vi "RL-Spect-Fast.vi"() -> ()   [LabVIEW 2014]
doc: "Random Laser Project\n\nAndré Romero - 2020\nandretec@ifsc.usp.br\n\nMain Program"
uses:
  Global variables.vi
panel:
  in  "Integration Time":i32=100
  in  "Average":i32=1
  out "Delay Power Meter":u32
  out "Delay Spectrum":u32
  in  "Stop Button":bool
  out "Power":dbl
  in  "Average Time (0.0)":dbl=0.1
  out "XY Graph":T1(graph)
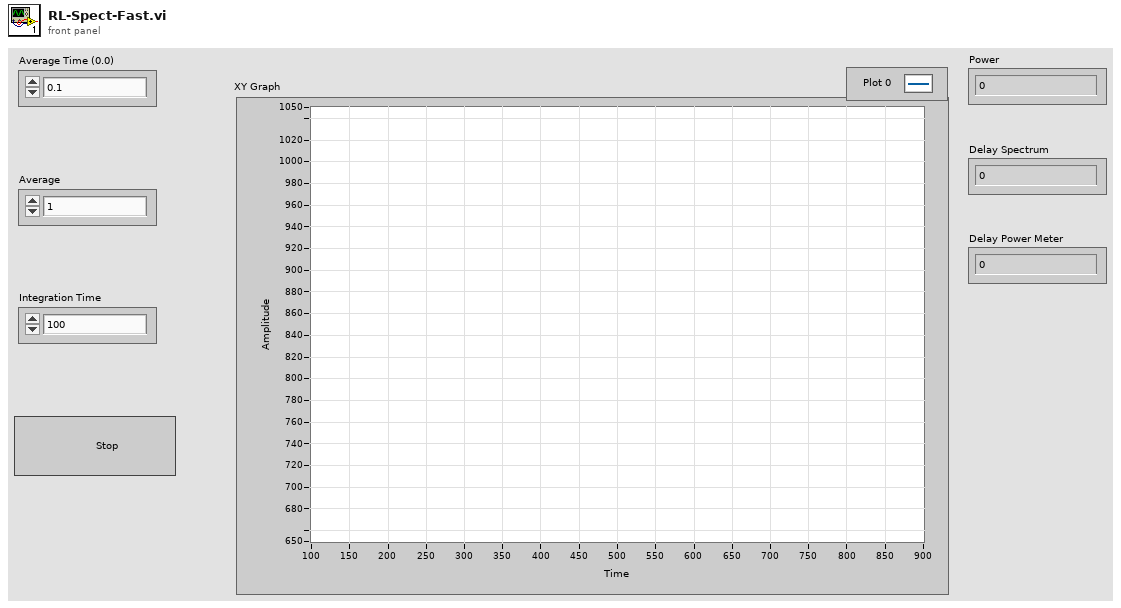
[diagram p1: front panel]
types:
  T1 = cluster{"WL Values":dbl[], "Spectrum Values":dbl[]}
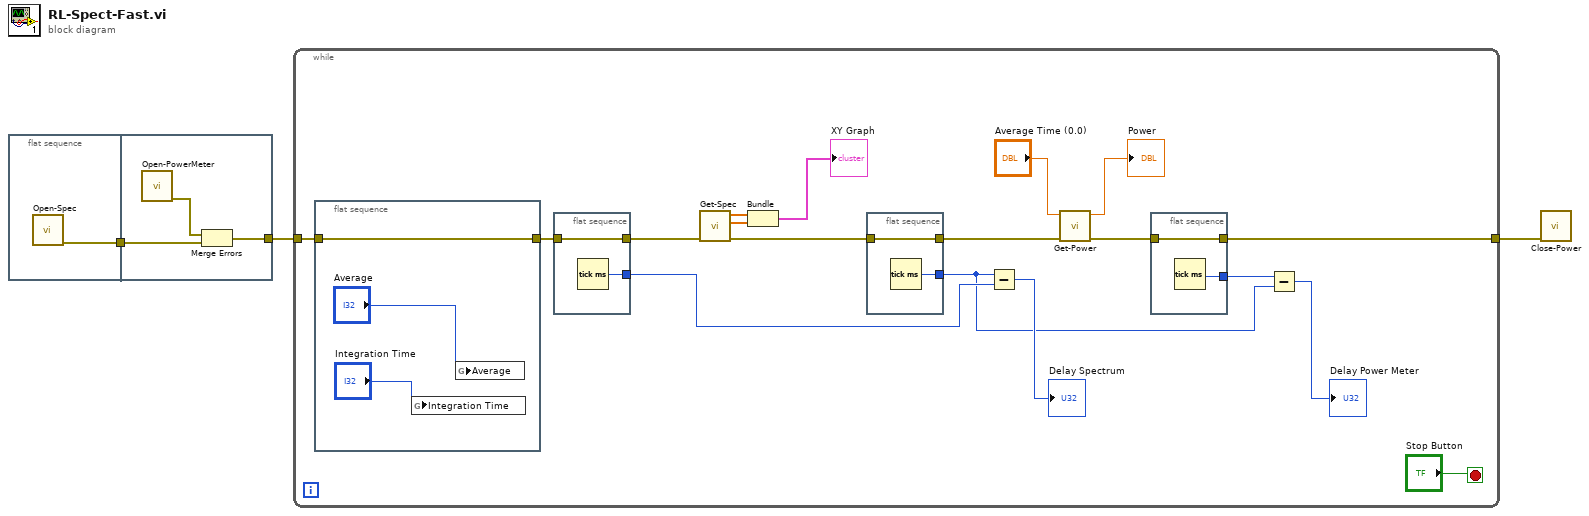
[diagram p0: block diagram]
diagram:
  n1 = flat-sequence {
    tunnel: [w4] -> w3
    tunnel: w3 -> [w6]
    tunnel: [w5] -> w2
    frame #0 {
      n2 = call "Open-Spec.vi"() -> ("error out"=w4:errorcluster)  [unwired: 9 in, 2 out]
    }
    frame #1 {
      n3 = call "Open-PowerMeter.vi"() -> ("error out"=w7:errorcluster)  [unwired: 10 in, 1 out]
      n4 = Merge Errors(w7, w6) -> (w5:errorcluster)
    }
  }
  n5 = while {
    tunnel: w2 -> [w9]
    tunnel: [w16] -> w1
    stop <- "Stop Button" stop-if-true
    n6 = flat-sequence {
      tunnel: w9 -> [w26]
      tunnel: [w26] -> w8
      frame #0 {
        n7 = global write "Global variables.vi" "Integration Time"("Integration Time") -> ()
        n8 = global write "Global variables.vi" "Average"("Average") -> ()
      }
    }
    n9 = flat-sequence {
      tunnel: w8 -> [w34]
      tunnel: [w34] -> w20
      tunnel: [w33] -> w14
      frame #0 {
        n10 = Tick Count (ms)() -> (millisecond timer value=w33:u32)
      }
    }
    n11 = call "Get-Spec.vi"("Error In"=w20) -> ("Error Out"=w19:errorcluster, "Spectrum Values"=w24:dbl[], "WL Values"=w25:dbl[])  [unwired: 8 in]
    n12 = Bundle("WL Values"=w25, "Spectrum Values"=w24) -> (→"XY Graph":T1)  [unwired: 1 in]
    n13 = flat-sequence {
      tunnel: w19 -> [w32]
      tunnel: [w32] -> w18
      tunnel: [w31] -> w11
      frame #0 {
        n14 = Tick Count (ms)() -> (millisecond timer value=w31:u32)
      }
    }
    n15 = Subtract(x=w11, y=w14) -> (x-y=→"Delay Spectrum":u32)
    n16 = call "Get-Power.vi"("error in"=w18, "Average Time (0.0)"="Average Time (0.0)") -> ("error out"=w17:errorcluster, "Power"=→"Power":dbl)  [unwired: 8 in]
    n17 = flat-sequence {
      tunnel: w17 -> [w30]
      tunnel: [w30] -> w16
      tunnel: [w29] -> w12
      frame #0 {
        n18 = Tick Count (ms)() -> (millisecond timer value=w29:u32)
      }
    }
    n19 = Subtract(x=w12, y=w11) -> (x-y=→"Delay Power Meter":u32)
  }
  n20 = call "Close-Power.vi"("error in (no error)"=w1) -> ()  [unwired: 11 in]
